vi "V7310.Status.Get.vi"(6 "timeout ms (5000)":i32=5000, 8 "error in":errorcluster, 11 "Connection in":refnum<k5>) -> (0 "error out":errorcluster, 1 "Laser Status":string, 2 "LaserStatus":T1, 3 "Connection out":refnum<k5>)   [LabVIEW 2016]
uses:
  LowLevel/V7310.LaserStatus.ctl
  LowLevel/V7310.Commands.ctl
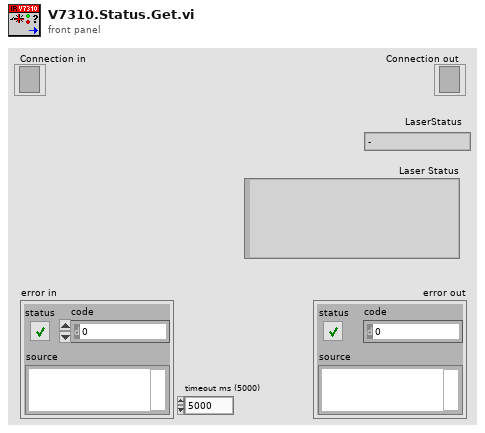
[diagram p1: front panel]
types:
  T1 = typedef "V7310.LaserStatus.ctl" = enum16{"-", "FatalError", "Initialize", "KeySwitchOpen", "TimeoutInterlock", "InterlockOpen", "StartUp", "ShutterlockOpen", "Standby", "Ready", "PrepareForMarking", "WaitForTrigger", "Marking"}
  T2 = typedef "V7310.Commands.ctl" = enum16{"Start", "Stop", "GetStatus", "GetVarNames", "GetJobNames", "SetJob", "GetJob", "SetVars", "GetVars", "SetLayoutPosition", "SetRotation", "GetMessageID", "GetMessages", "ConfirmMessages", "DeleteMessages", "SetRTC", "GetRTC", "SetVarPosition", "SetIntensity", "GetIntensity", "SetStartTriggerDelay", "GetStartTriggerDelay", "SetStopTriggerDelay", "GetStopTriggerDelay", "SetConsecutiveTriggerDelay", "GetConsecutiveTriggerDelay", "SetMarkSpeed", "GetMarkSpeed"}
  T3 = typedef "V7310.ErrorLevels.ctl" = enum16{"OK", "Warning", "Error"}
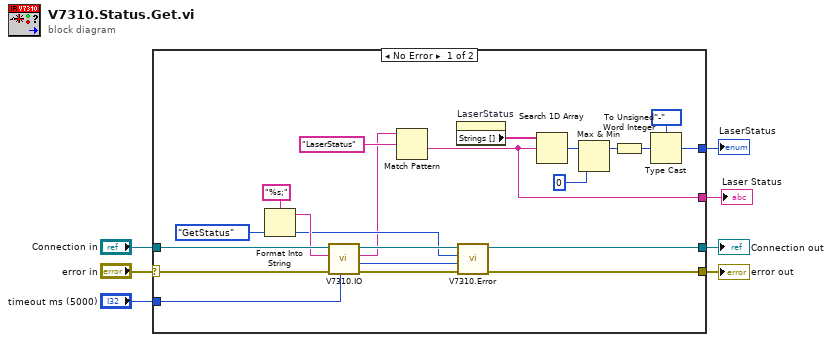
[diagram p0: block diagram]
diagram:
  n1 = case shown="No Error" "error in" {
    selector: "error in" -> [w25 w28]
    tunnel: "Connection in" -> [w26 w29]
    tunnel: [w27 w29] -> w6
    tunnel: "timeout ms (5000)" -> [w24 _]
    tunnel: [w23 w28] -> w3
    tunnel: [w22 _] -> w2
    tunnel: [w21 _] -> w1
    frame No Error {
      w18 = V7310.Commands."GetStatus" ("Cmd")
      n2 = Format Into String(format string="%s;", w18) -> (resulting string=w19:string)  [unwired: 2 in, 1 out]
      n3 = call "V7310.IO.vi"("timeout ms (5000)"=w24, "error in"=w25, "Data in"=w19, "Connection in"=w26) -> ("error out"=w16:errorcluster, "Error Level"=w17:T3, "Data out"=w9:string, "Connection out"=w27:refnum<k5>)  [unwired: 4 in]
      n4 = Match Pattern(string=w9, regular expression="LaserStatus" ("search string")) -> (after substring=w21:string)  [unwired: 1 in, 3 out]
      n5 = property on="LaserStatus" class="Enum (strict)"() -> ("Strings []"=w14:string[])  [unwired: 2 in, 2 out]
      n6 = call "V7310.Error.vi"("error in"=w16, "Error Level"=w17, "Cmd"=w18) -> ("error out"=w23:errorcluster)  [unwired: 8 in]
      n7 = Search 1D Array(1D array=w14, element=w21) -> (index of element=w12:i32)  [unwired: 1 in]
      n8 = Max & Min(x=w12, y=0) -> (max(x,y)=w10:i32)  [unwired: 1 out]
      n9 = To Unsigned Word Integer(number=w10) -> (unsigned 16bit integer=w8:u16)
      n10 = Type Cast(type=V7310.LaserStatus."-" ("LaserStatus"), x=w8) -> (*(type *) &x=w22:T1)
    }
    frame Error {
    }
  }
  "Connection out" <- w6
  "error out" <- w3
  "LaserStatus" <- w2
  "Laser Status" <- w1
